vi "Excel_TrippedTime.vi"(6 "1_IL,0_uL":bool, 7 "Result":cluster{"Tripped Time":i32[], "KGR":dbl[]}, 8 "error in (no error)":errorcluster, 9 "Test?":bool, 10 "Report path in":path, 11 "report in":refnum<class "NI_report.lvclass">) -> (0 "error out":errorcluster, 2 "Report path out":path, 3 "report out":refnum<class "NI_report.lvclass">)   [LabVIEW 2015]
doc: "输出uL,IL的\n脱扣时间和电路因子"
uses:
  <vilib>/Utility/NIReport.llb/NI_report.lvclass
  <vilib>/addons/_office/NI_ReportGenerationToolkit.lvlib
panel:
  in  "start(-1,-1)":cluster{"row":i32, "column":i32}
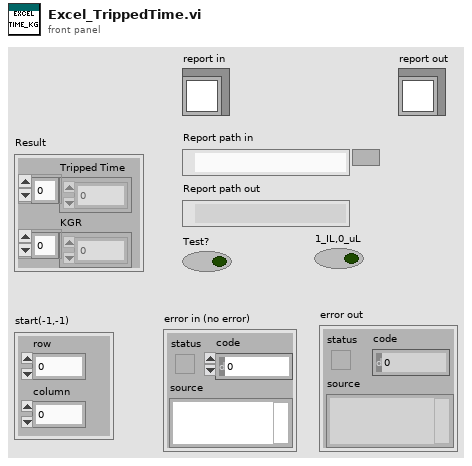
[diagram p1: front panel]
types:
  T1 = enum16{"Standard Report", "HTML", "Word", "Excel"}
  T2 = enum16{"maximized", "minimized", "normal", "no change"}
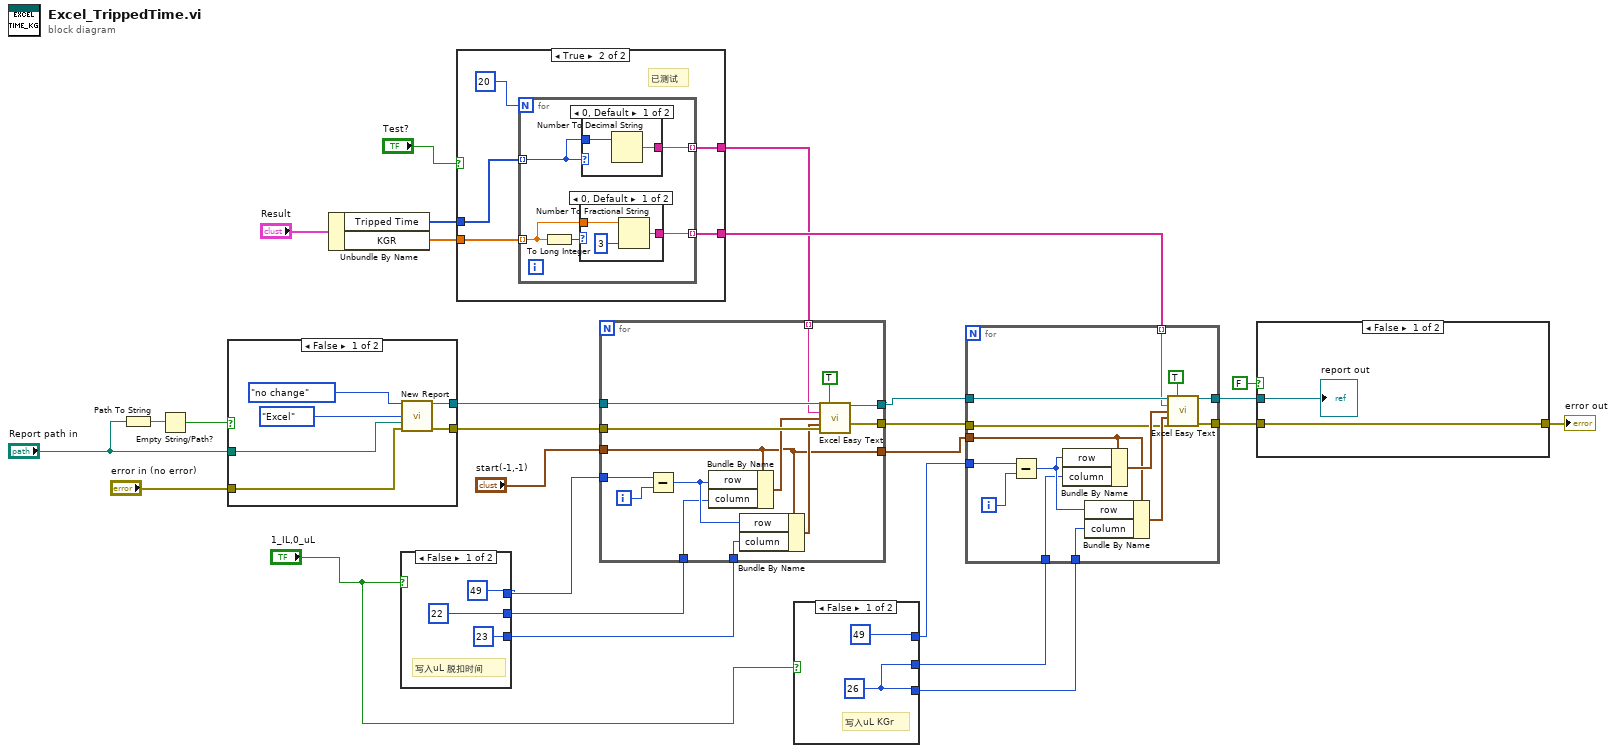
[diagram p0: block diagram]
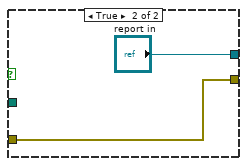
[diagram p2: hidden frame]
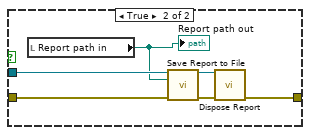
[diagram p3: hidden frame]
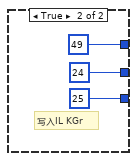
[diagram p4: hidden frame]
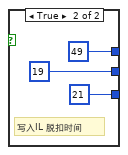
[diagram p5: hidden frame]
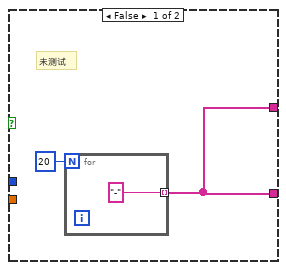
[diagram p6: hidden frame]
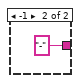
[diagram p7: hidden frame]
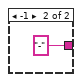
[diagram p8: hidden frame]
diagram:
  n1 = Path To String(path="Report path in") -> (string=w3:string)
  n2 = Empty String/Path?(string/path=w3) -> (empty?=w2:bool)
  n3 = case shown="False" w2 {
    tunnel: [w33 "report in"] -> w23
    tunnel: [w32 w35] -> w22
    tunnel: "error in (no error)" -> [w29 w35]
    tunnel: "Report path in" -> [w28 _]
    frame False {
      n4 = call <vilib>:"New Report.vi"("window state (normal)"=T2."no change", "report type"=T1."Excel", "template (empty)"=w28, "error in (no error)"=w29) -> ("report out"=w33:refnum<class "NI_report.lvclass">, "error out"=w32:errorcluster)  [unwired: 10 in]
    }
    frame True {
    }
  }
  n5 = Unbundle By Name("Result") -> ("Tripped Time"=w1:i32[], "KGR"=w26:dbl[])
  n6 = case shown="False" "1_IL,0_uL" {
    tunnel: [49 ("x") 49 ("x")] -> w17
    tunnel: [22 ("x") 19 ("x")] -> w16
    tunnel: [23 21] -> w15
    frame False {
      # "写入uL 脱扣时间"
    }
    frame True {
      # "写入IL 脱扣时间"
    }
  }
  n7 = case shown="True" "Test?" {
    tunnel: w26 -> [_ w46]
    tunnel: [w42 w49] -> w25
    tunnel: [w42 w48] -> w24
    tunnel: w1 -> [_ w47]
    frame False {
      # "未测试"
      n8 = for {
        N: 20 -> [_]
        tunnel: ["-"] -> w42 mode=indexing
      }
    }
    frame True {
      # "已测试"
      n9 = for {
        N: 20 -> [_]
        tunnel: [w54] -> w49 mode=indexing
        tunnel: [w53] -> w48 mode=indexing
        tunnel: w47 -> [w52] mode=indexing
        tunnel: w46 -> [w51] mode=indexing
        n10 = To Long Integer(number=w51) -> (32bit integer=w50:i32)
        n11 = case shown="0, Default" w50 {
          tunnel: [w60 "-"] -> w54
          tunnel: w51 -> [w58 _]
          frame 0, Default {
            n12 = Number To Fractional String(number=w58, precision (6)=i16 3) -> (F-format string=w60:string)  [unwired: 2 in]
          }
          frame -1 {
          }
        }
        n13 = case shown="0, Default" w52 {
          tunnel: [w56 "-"] -> w53
          tunnel: w52 -> [w55 _]
          frame 0, Default {
            n14 = Number To Decimal String(number=w55) -> (decimal integer string=w56:string)  [unwired: 1 in]
          }
          frame -1 {
          }
        }
      }
    }
  }
  n15 = for {
    tunnel: w23 -> [w75]
    tunnel: w22 -> [w74]
    tunnel: [w73] -> w20
    tunnel: [w72] -> w19
    tunnel: "start(-1,-1)" -> [w65]
    tunnel: w24 -> [w66] mode=indexing
    tunnel: [w65] -> w18
    tunnel: w17 -> [w64]
    tunnel: w16 -> [w63]
    tunnel: w15 -> [w62]
    i -> [w68]
    n16 = Subtract(x=w64, y=w68) -> (x-y=w69:i32)
    n17 = Bundle By Name(cluster=w65, "row"=w69, "column"=w63) -> (w71:cluster{"row":i32, "column":i32})
    n18 = Bundle By Name(cluster=w65, "row"=w69, "column"=w62) -> (w70:cluster{"row":i32, "column":i32})
    n19 = call <vilib>:"Excel Easy Text.vi"("report in"=w75, "border? (F)"=TRUE, "text"=w66, "start (-1, -1)"=w71, "end (-1, -1)"=w70, "error in (no error)"=w74) -> ("report out"=w73:refnum<class "NI_report.lvclass">, "error out"=w72:errorcluster)  [unwired: 5 in, 3 out]
  }
  n20 = case shown="False" "1_IL,0_uL" {
    tunnel: [49 ("row") 49 ("row")] -> w14
    tunnel: [w76 24 ("column")] -> w13
    tunnel: [w76 25 ("column")] -> w12
    frame False {
      w76 = 26 ("column")
      # "写入uL KGr"
    }
    frame True {
      # "写入IL KGr"
    }
  }
  n21 = for {
    tunnel: w18 -> [w89]
    tunnel: w20 -> [w88]
    tunnel: w19 -> [w87]
    tunnel: [w86] -> w9
    tunnel: [w85] -> w8
    tunnel: w25 -> [w84] mode=indexing
    tunnel: w14 -> [w83]
    tunnel: w13 -> [w82]
    tunnel: w12 -> [w81]
    i -> [w90]
    n22 = Subtract(x=w83, y=w90) -> (x-y=w94:i32)
    n23 = Bundle By Name(cluster=w89, "row"=w94, "column"=w82) -> (w92:cluster{"row":i32, "column":i32})
    n24 = Bundle By Name(cluster=w89, "row"=w94, "column"=w81) -> (w93:cluster{"row":i32, "column":i32})
    n25 = call <vilib>:"Excel Easy Text.vi"("report in"=w88, "border? (F)"=TRUE, "text"=w84, "start (-1, -1)"=w92, "end (-1, -1)"=w93, "error in (no error)"=w87) -> ("report out"=w86:refnum<class "NI_report.lvclass">, "error out"=w85:errorcluster)  [unwired: 5 in, 3 out]
  }
  n26 = case shown="False" FALSE {
    tunnel: [w96 w102] -> w10
    tunnel: w9 -> [w95 w99]
    tunnel: w8 -> [w96 w98]
    frame False {
      "report out" <- w95
    }
    frame True {
      n27 = local read "Report path in"() -> (w97:path)
      "Report path out" <- w97
      n28 = call-dynamic "Save Report to File.vi"("report in"=w99, "report file path"=w97, "error in (no error)"=w98) -> ("report out"=w100:refnum<class "NI_report.lvclass">, "error out"=w101:errorcluster)  [unwired: 11 in]
      n29 = call-dynamic "Dispose Report.vi"("report in"=w100, "error in (no error)"=w101) -> ("error out"=w102:errorcluster)  [unwired: 13 in]
    }
  }
  "error out" <- w10
